vi "Copy_with_Check.vi"(1 "Mode":enum16{"Move", "Copy"}(ring)=enum."Copy", 2 "Target Path":path, 3 "Variable Target?":bool, 4 "Source Path":path) -> (0 "Pathname Out":path)   [LabVIEW 2022 SP3]
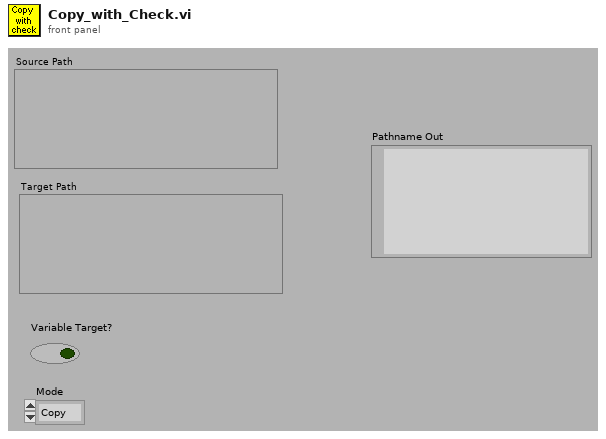
[diagram p1: front panel]
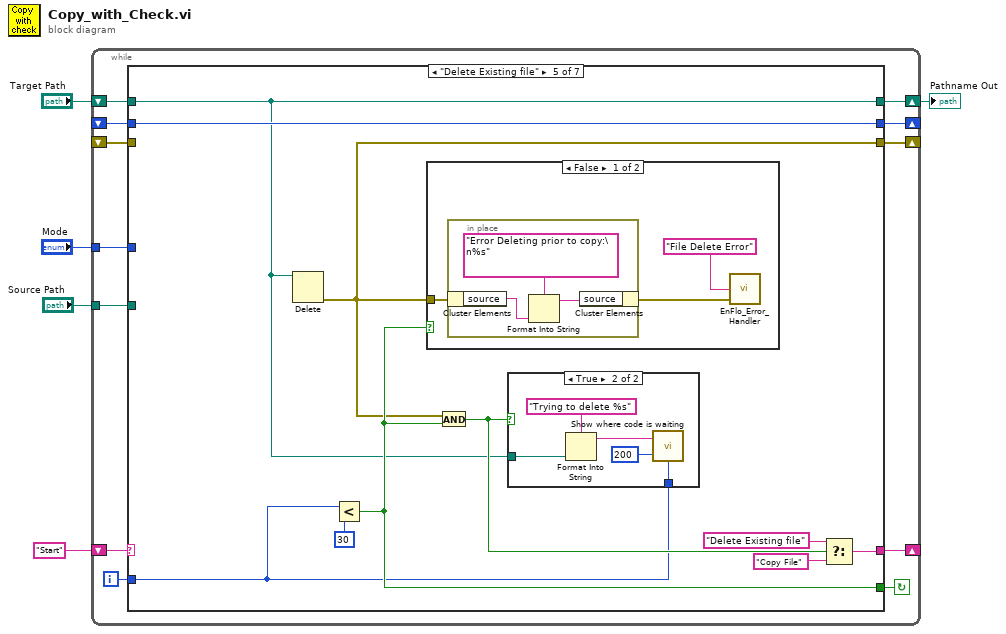
[diagram p0: block diagram]
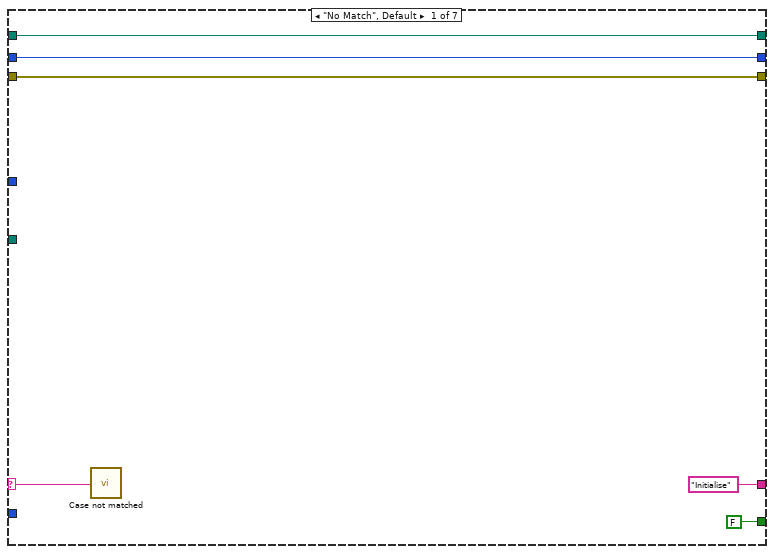
[diagram p2: hidden frame]
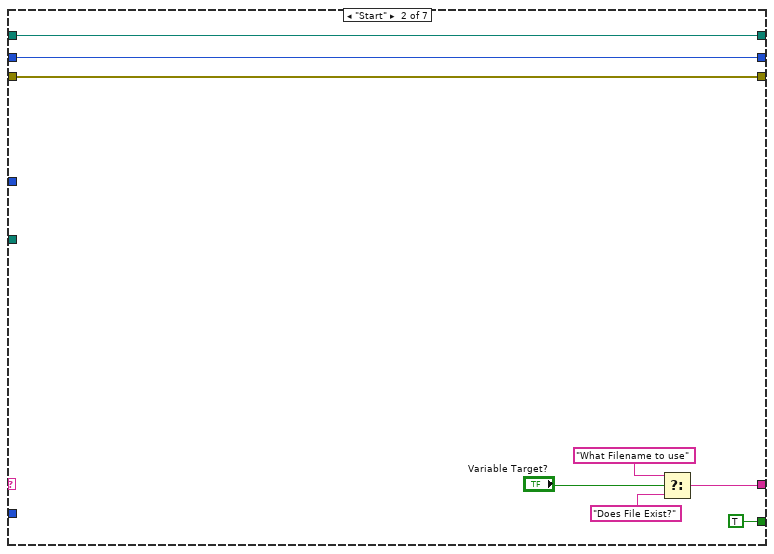
[diagram p3: hidden frame]
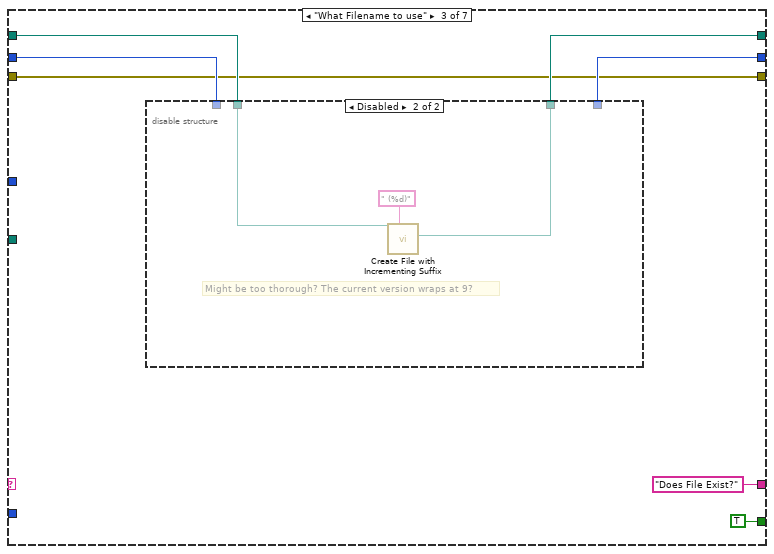
[diagram p4: hidden frame]
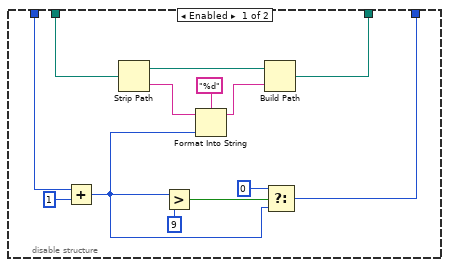
[diagram p5: hidden frame]
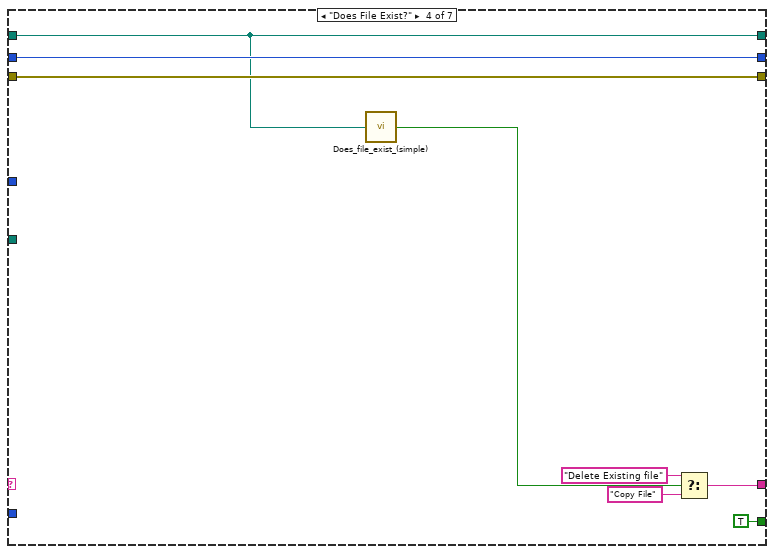
[diagram p6: hidden frame]
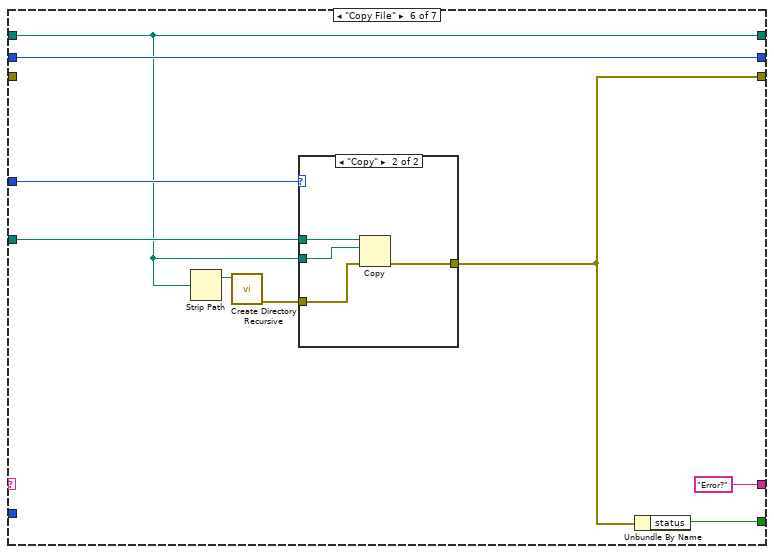
[diagram p9: hidden frame]
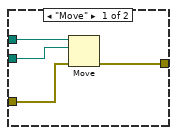
[diagram p10: hidden frame]
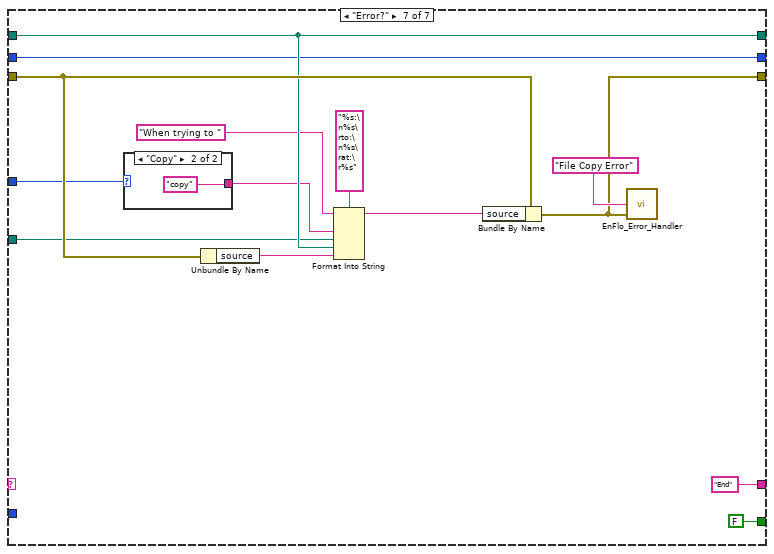
[diagram p11: hidden frame]
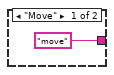
[diagram p12: hidden frame]
diagram:
  n1 = while {
    shift-left: "Start" -> [w15]
    shift-right: [w16] -> _
    shift-right: [w11] -> w3
    shift-left: "Target Path" -> [w14]
    shift-right: [w12] -> _
    shift-left: _ -> [w13]
    shift-right: [w10] -> _
    shift-left: _ -> [w9]
    tunnel: "Source Path" -> [w8]
    tunnel: "Mode" -> [w6]
    i -> [w7]
    stop <- w17 continue-if-true
    n2 = case shown="\"Delete Existing file\"" w15 {
      selector: w15 -> [w18 _ _ _ _ _ _]
      tunnel: [FALSE TRUE TRUE TRUE w66 w87 FALSE] -> w17
      tunnel: ["Initialise" w28 "Does File Exist?" ("f") w60 w72 "Error?" "End"] -> w16
      tunnel: w14 -> [w21 w30 w36 w56 w63 w85 w108]
      tunnel: w13 -> [w20 w25 w37 w57 w70 w89 w107]
      tunnel: [w20 w25 w35 w57 w70 w89 w107] -> w12
      tunnel: [w21 w30 w34 w56 w63 w85 w108] -> w11
      tunnel: [w19 w24 w32 w58 w65 w91 w106] -> w10
      tunnel: w9 -> [w19 w24 w32 w58 _ _ w110]
      tunnel: w8 -> [_ _ _ _ _ w90 w103]
      tunnel: w7 -> [_ _ _ _ w64 _ _]
      tunnel: w6 -> [_ _ _ _ _ w88 w105]
      frame "No Match", Default {
        n3 = call "Case not matched.vi"("Case Name not Matched"=w18) -> ()
      }
      frame "Start" {
        n4 = Select(t="What Filename to use", s="Variable Target?", f="Does File Exist?") -> (s? t:f=w28:string)
      }
      frame "What Filename to use" {
        n5 = disable-structure shown="Disabled" {
          disable-tunnel: w37 -> [w51 _]
          disable-tunnel: w36 -> [w49 w54]
          disable-tunnel: [w40 _] -> w35
          disable-tunnel: [w39 w53] -> w34
          frame Enabled {
            n6 = Add(x=w51, y=1) -> (x+y=w42:i32)
            n7 = Strip Path(path=w49) -> (stripped path=w46:path, name=w48:string)
            n8 = Greater?(x=w42, y=9) -> (0:w43:bool)
            n9 = Format Into String(format string="%d", initial string=w48, w42) -> (resulting string=w45:string)  [unwired: 1 in, 1 out]
            n10 = Build Path(base path=w46, name or relative path=w45) -> (appended path=w39:path)
            n11 = Select(t=0, s=w43, f=w42) -> (s? t:f=w40:i32)
          }
          frame Disabled {
            # "Might be too thorough? The current version wraps at 9?"
            n12 = call <vilib>:"Create File with Incrementing Suffix.vi"("format string (\" (%d)\")"=" (%d)" ("format string (\" (%d)\")"), "file path"=w54) -> ("actual path"=w53:path)  [unwired: 7 in, 2 out]
          }
        }
      }
      frame "Does File Exist?" {
        n13 = call "Does_file_exist_(simple).vi"("Pathname"=w56) -> ("exists?"=w61:bool)
        n14 = Select(t="Delete Existing file", s=w61, f="Copy File") -> (s? t:f=w60:string)
      }
      frame "Delete Existing file" {
        n15 = Delete(path (use dialog)=w63) -> (error out=w65:errorcluster)  [unwired: 1 in, 5 out]
        n16 = Less?(x=w64, y=30) -> (x < y?=w66:bool)
        n17 = case shown="False" w66 {
          tunnel: w65 -> [w74 _]
          frame False {
            n18 = in-place {
              n19 = in-place-cluster #1(w74) -> ("source"=w77:string)
              n20 = Format Into String(format string="Error Deleting prior to copy:\n%s", w77) -> (resulting string=w76:string)  [unwired: 2 in, 1 out]
              n21 = in-place-cluster #1("source"=w76) -> (w73:errorcluster)
            }
            n22 = call "EnFlo_Error_Handler.vi"("error in (no error)"=w73, "Error Type"="File Delete Error") -> ()  [unwired: 1 in, 3 out]
          }
          frame True {
          }
        }
        n23 = And(x=w65, y=w66) -> (x .and. y?=w68:bool)
        n24 = case shown="True" w68 {
          tunnel: w64 -> [_ w82]
          tunnel: w63 -> [_ w81]
          frame False {
          }
          frame True {
            n25 = Format Into String(format string="Trying to delete %s", w81) -> (resulting string=w79:string)  [unwired: 2 in, 1 out]
            n26 = call "Show where code is waiting.vi"("Loop index"=w82, "Wait (ms)"=u32 200 ("milliseconds to wait"), "Message"=w79) -> ()  [unwired: 1 in]
          }
        }
        n27 = Select(t="Delete Existing file", s=w68, f="Copy File") -> (s? t:f=w72:string)
      }
      frame "Copy File" {
        n28 = Strip Path(path=w85) -> (stripped path=w86:path)  [unwired: 1 out]
        n29 = call <vilib>:"Create Directory Recursive.vi"("directory"=w86) -> ("error out"=w84:errorcluster)  [unwired: 4 in, 2 out]
        n30 = case shown="\"Copy\"" w88 {
          tunnel: [w94 w100] -> w91
          tunnel: w90 -> [w96 w99]
          tunnel: w85 -> [w95 w98]
          tunnel: w84 -> [w93 w97]
          frame "Move" {
            n31 = Move(source path=w96, error in=w93, 10:w95) -> (error out=w94:errorcluster)  [unwired: 4 out]
          }
          frame "Copy" {
            n32 = Copy(8:w97, 10:w98, 11:w99) -> (0:w100:errorcluster)  [unwired: 4 out]
          }
        }
        n33 = Unbundle By Name(w91) -> ("status"=w87:bool)
      }
      frame "Error?" {
        n34 = case shown="\"Copy\"" w105 {
          tunnel: ["move" ("format string") "copy" ("format string")] -> w102
          frame "Move" {
          }
          frame "Copy" {
          }
        }
        n35 = Unbundle By Name(w110) -> ("source"=w111:string)
        n36 = Format Into String(format string="%s:\n%s\rto:\n%s\rat:\r%s", initial string="When trying to " ("format string"), w102, w103, w108, w111) -> (resulting string=w109:string)  [unwired: 1 in, 1 out]
        n37 = Bundle By Name(cluster=w110, "source"=w109) -> (w106:errorcluster)
        n38 = call "EnFlo_Error_Handler.vi"("error in (no error)"=w106, "Error Type"="File Copy Error") -> ()  [unwired: 1 in, 3 out]
      }
    }
  }
  "Pathname Out" <- w3
